vi "Add to Tree.vi"(4 "Child Tag":string, 5 "Child Position":i32, 6 "Display Text Override":string, 7 "Add children? (T)":bool=TRUE, 8 "error in (no error)":errorcluster, 9 "Parent Tag":string, 10 "Tree Manager in":refnum<class "Tree Manager.lvclass">, 11 "Attribute in":refnum<class "Attribute.lvclass">) -> (0 "error out":errorcluster, 2 "Tree Manager out":refnum<class "Tree Manager.lvclass">, 3 "Attribute out":refnum<class "Attribute.lvclass">)   [LabVIEW 2026, in "VILab.lvlib" / "Attribute.lvclass"]
uses:
  Attribute.lvclass
  Tree Manager/Tree Manager.lvclass
  Data Item/Data Item.lvclass
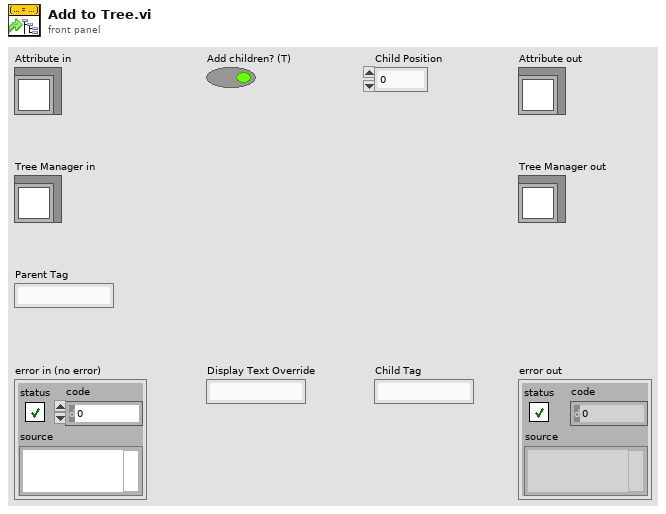
[diagram p1: front panel]
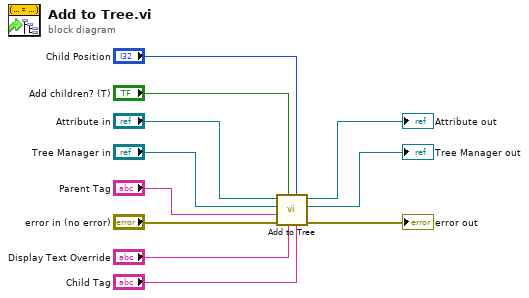
[diagram p0: block diagram]
diagram:
  n1 = call-parent "Add to Tree.vi"("Child Tag"="Child Tag", "Child Position"="Child Position", "Display Text Override"="Display Text Override", "Add children? (T)"="Add children? (T)", "error in (no error)"="error in (no error)", "Parent Tag"="Parent Tag", "Tree Manager in"="Tree Manager in", "Data Item in"="Attribute in") -> ("error out"=→"error out":errorcluster, "Tree Manager out"=→"Tree Manager out":refnum<class "Tree Manager.lvclass">, "Data Item out"=→"Attribute out":refnum<class "Attribute.lvclass">)  [unwired: 1 in]
